vi "Save Settings Section.vi"(8 "Error in":errorcluster caption="Error in (no error)", 9 "JSON Object":string, 10 "Section Name":string, 11 "JSON Settings Path":path) -> (0 "Error out":errorcluster)   [LabVIEW 2023, in "VIDoc Settings.lvclass"]
uses:
  VIDoc Settings.lvclass
  <vilib>/JDP Science/JSONtext/JSONtext.lvlib
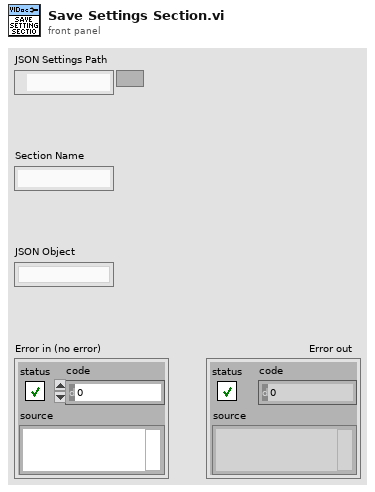
[diagram p1: front panel]
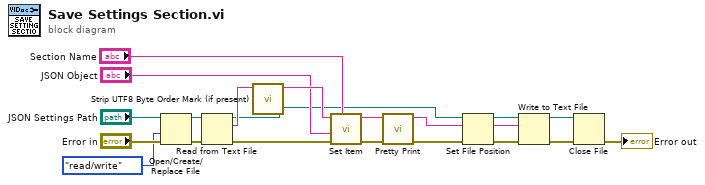
[diagram p0: block diagram]
diagram:
  n1 = Open/Create/Replace File(file path (use dialog)="JSON Settings Path", error in="Error in", access (0:read/write)=enum16{"read/write", "read-only", "write-only"}."read/write") -> (refnum out=w16:refnum<file>, error out=w17:errorcluster)  [unwired: 3 in, 1 out]
  n2 = Read from Text File(file (use dialog)=w16, error in=w17) -> (refnum out=w4:refnum<file>, text=w15:string, error out=w11:errorcluster)  [unwired: 2 in, 1 out]
  n3 = call <vilib>:"Strip UTF8 Byte Order Mark (if present).vi"("Text in"=w15) -> ("Possible Byte Order Mark Stripped"=w14:string)  [unwired: 9 in, 1 out]
  n4 = call <vilib>:"Set Item.vi"("$Path or Item Name"="Section Name", "error in (no error)"=w11, "JSON to Insert"="JSON Object", "JSON"=w14) -> ("error out"=w6:errorcluster, "<JSON>"=w7:string)  [unwired: 4 in, 1 out]
  n5 = call <vilib>:"Pretty Print.vi"("error in (no error)"=w6, "JSON"=w7) -> ("error out"=w3:errorcluster, "<JSON>"=w5:string)  [unwired: 7 in, 1 out]
  n6 = Set File Position(refnum=w4, error in=w3) -> (refnum out=w1:refnum<file>, error out=w2:errorcluster)  [unwired: 2 in]
  n7 = Write to Text File(file (use dialog)=w1, text=w5, error in=w2) -> (refnum out=w10:refnum<file>, error out=w9:errorcluster)  [unwired: 1 in, 1 out]
  n8 = Close File(refnum=w10, error in=w9) -> (error out=→"Error out":errorcluster)  [unwired: 1 out]
